vi "Split 1D Array.vi"(5 "JSON Array":refnum<class "JSON Array.lvclass">, 9 "index":i32) -> (6 "first subarray":refnum<class "JSON Array.lvclass">, 10 "second subarray":refnum<class "JSON Array.lvclass">)   [LabVIEW 2015, in "LVJSON.lvlib" / "JSON Array.lvclass"]
doc: "Divides array at index and returns the two portions with the element of index at the beginning of second subarray."
uses:
  JSON Array.lvclass
  JSON Array.lvclass/JSON Array.ctl
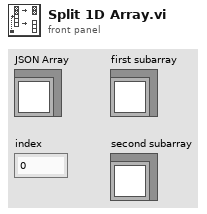
[diagram p1: front panel]
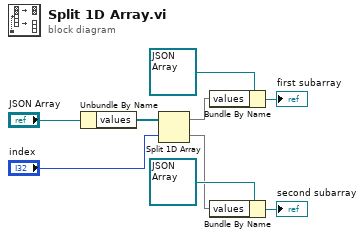
[diagram p0: block diagram]
diagram:
  n1 = Unbundle By Name("JSON Array") -> ("values"=w1:refnum<class "JSON Null.lvclass">[])
  n2 = Split 1D Array(array=w1, index="index") -> (first subarray=w3:refnum<class "JSON Null.lvclass">[], second subarray=w2:refnum<class "JSON Null.lvclass">[])
  n3 = Bundle By Name(cluster=refnum<class "JSON Array.lvclass"> refnum ("JSON Array"), "values"=w3) -> (→"first subarray":refnum<class "JSON Array.lvclass">)
  n4 = Bundle By Name(cluster=refnum<class "JSON Array.lvclass"> refnum ("JSON Array"), "values"=w2) -> (→"second subarray":refnum<class "JSON Array.lvclass">)
